vi "OPO_TCP_Client_Ack.vi"(8 "error in (no error)":errorcluster, 10 "ACK letter":string="Q", 11 "TCP Network Connection in":refnum<k5>) -> (0 "error out":errorcluster, 3 "bytes written":i32)   [LabVIEW 2020]
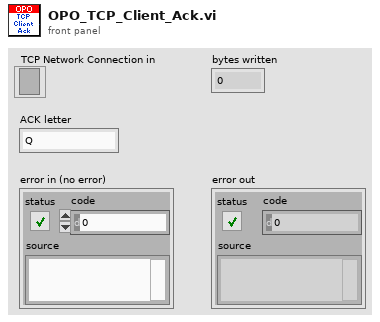
[diagram p1: front panel]
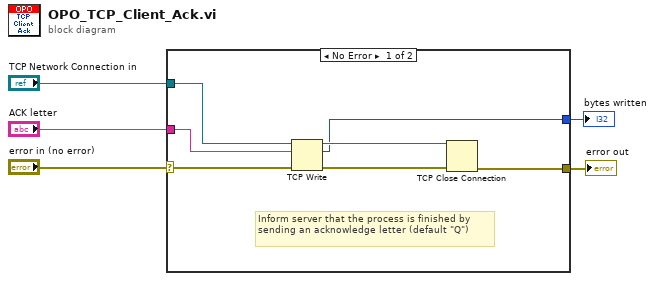
[diagram p0: block diagram]
diagram:
  n1 = case shown="No Error" "error in (no error)" {
    selector: "error in (no error)" -> [w7 w13]
    tunnel: "ACK letter" -> [w12 _]
    tunnel: "TCP Network Connection in" -> [w9 _]
    tunnel: [w8 w13] -> w3
    tunnel: [w6 _] -> w1
    frame No Error {
      # "Inform server that the process is finished by sending an acknowledge letter (default \"Q\")"
      n2 = TCP Write(connection ID=w9, data in=w12, error in (no error)=w7) -> (connection ID out=w10:refnum<k5>, bytes written=w6:i32, error out=w11:errorcluster)  [unwired: 1 in]
      n3 = TCP Close Connection(connection ID=w10, error in (no error)=w11) -> (error out=w8:errorcluster)  [unwired: 1 in, 1 out]
    }
    frame Error {
    }
  }
  "error out" <- w3
  "bytes written" <- w1
